vi "Get Std Devs.vi"(7 "ChunkSize":i32[](array[numeric])=[5, 10, 25, 50, 100, 250], 11 "DataIn":dbl[](array[numeric])) -> (3 "StdDevOut":sgl[](array[numeric]))   [LabVIEW 2014, in "CRDS Lib.lvlib" / "CRDS Cell.lvclass"]
uses:
  CRDS/Cell/CRDS Cell.lvclass
  <vilib>/Analysis/baseanly.llb/Mean (DBL).vi
  <vilib>/Analysis/NI_AALBase.lvlib
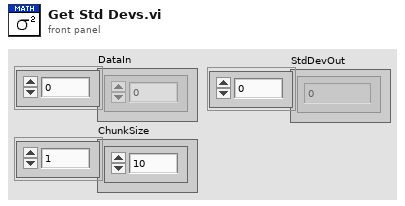
[diagram p1: front panel]
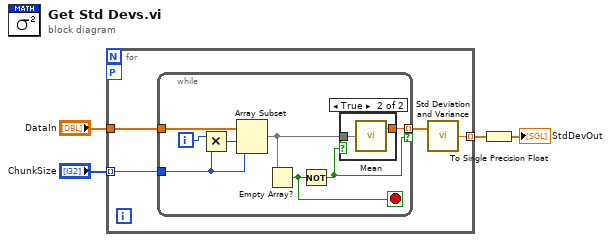
[diagram p0: block diagram]
diagram:
  n1 = for {
    tunnel: "ChunkSize" -> [w7] mode=indexing
    workers-P: _ -> [_]
    tunnel: "DataIn" -> [w8]
    tunnel: [w5] -> w2 mode=indexing
    n2 = while {
      tunnel: w7 -> [w14]
      tunnel: w8 -> [w16]
      tunnel: [w12] -> w6 mode=indexing if=w10
      i -> [w15]
      stop <- w9 stop-if-true
      n3 = Multiply(x=w15, y=w14) -> (x*y=w13:i32)
      n4 = Array Subset(array=w16, index=w13, length=w14) -> (w11:dbl[])
      n5 = Empty Array?(array=w11) -> (empty?=w9:bool)
      n6 = Not(x=w9) -> (.not. x?=w10:bool)
      n7 = case shown="True" w10 {
        tunnel: [_ w18] -> w12
        tunnel: w11 -> [_ w17]
        frame False {
        }
        frame True {
          n8 = call-poly <vilib>:"Mean.vi"("X"=w17) -> ("mean"=w18:dbl)  [unwired: 1 out]
        }
      }
    }
    n9 = call <vilib>:"Std Deviation and Variance.vi"("X"=w6) -> ("standard deviation"=w5:dbl)  [unwired: 1 in, 2 out]
  }
  n10 = To Single Precision Float(number=w2) -> (single precision float=→"StdDevOut":sgl[])
